vi "RUC_measurment(F-x).vi"() -> ()   [LabVIEW 2018]
panel:
  in  "Filename":path=path "C:/Users/Bizjan/Desktop/Structural dynamics of 3D printed thermoactive metamaterials/Measurements/RUC_measunments/test.lvm"
  out "F(x) [N/mm]":cluster{"Y":dbl[], "Y":dbl[]}[](graph)
  out "Pomik x [mm]":dynamicdata(graph)
  out "Sila F [N]":dynamicdata(graph)
  in  "Enable":bool=TRUE
  in  "stop (F)":bool
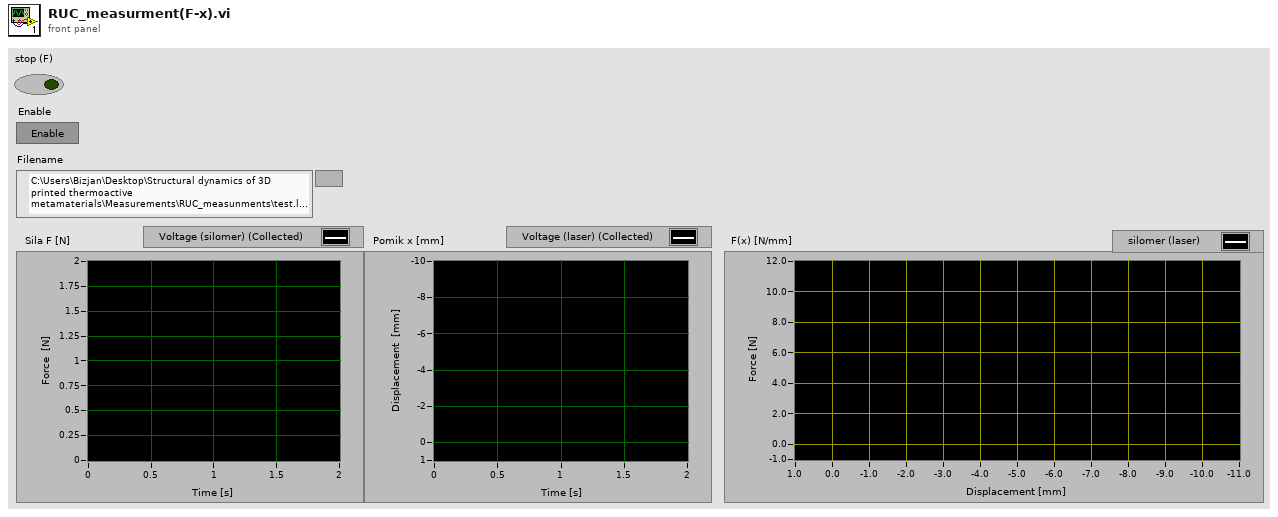
[diagram p1: front panel]
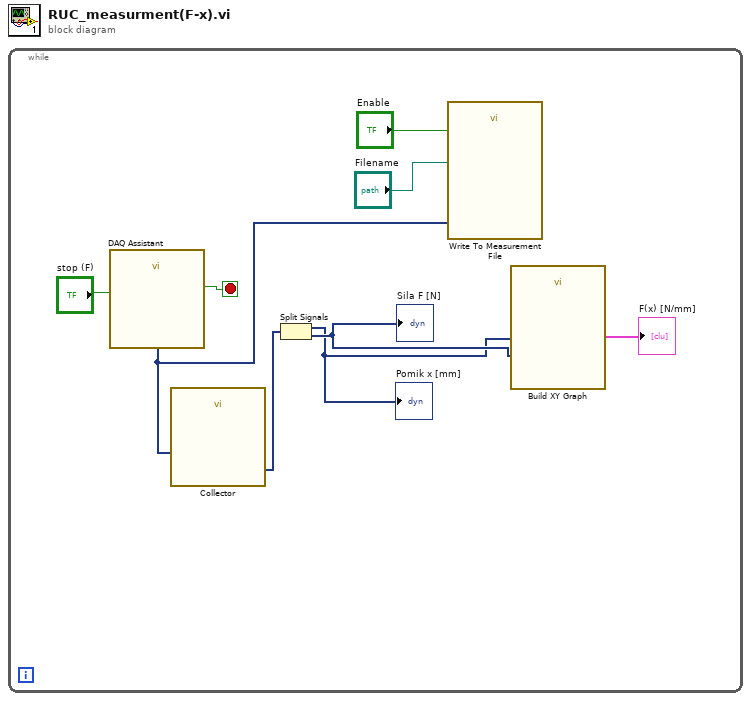
[diagram p0: block diagram]
diagram:
  n1 = while {
    stop <- w7 stop-if-true
    n2 = call "DAQ Assistant"("stop (F)"="stop (F)") -> ("data"=w2:dynamicdata, "stopped"=w7:bool)  [unwired: 15 in, 2 out]
    n3 = call "Collector"("Signals"=w2) -> ("Collected Signals"=w4:dynamicdata)  [unwired: 9 in, 1 out]
    n4 = Split Signals(w4) -> (w5:dynamicdata, w6:dynamicdata)  [unwired: 2 in]
    "Sila F [N]" <- w6
    "Pomik x [mm]" <- w5
    n5 = call "Write To Measurement File"("Signals"=w2, "Enable"="Enable", "Filename"="Filename") -> ()  [unwired: 14 in, 3 out]
    n6 = call "Build XY Graph"("Y Input"=w6, "X Input"=w5) -> ("XY Graph"=→"F(x) [N/mm]":cluster{"X":dbl[], "Y":dbl[]}[])  [unwired: 8 in, 1 out]
  }
